vi "save channels to raw bin files.vi"(8 "frame number in":i32, 9 "last frame":bool, 10 "image data in (SGL)":sgl[][](array[numeric]), 11 "image data in (U16)":u16[][](array[numeric])) -> ()   [LabVIEW 2012]
uses:
  Custom Controls/file format type def.ctl
  GFG/GFGpathGet.vi
  GFG/GFG library.lvlib
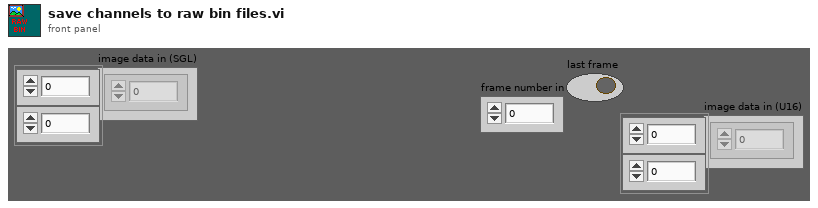
[diagram p1: front panel]
types:
  T1 = enum16{"open", "replace", "create", "open or create", "replace or create", "replace or create with confirmation"}
  T2 = typedef "file format type def.ctl" = enum16{"16bit raw", "32bit raw", "16bit multi-tiff (interleave)", "16bit multi-tiff (separate)", "16bit multi-tiff (stacked)", "32bit multi-tiff (interleave)", "32bit multi-tiff (separate)", "32bit multi-tiff (stacked)", "16bit tiff series (interleave)", "16bit tiff series (separate)", "16bit tiff series (stacked)", "32bit tiff series (interleave)", "32bit tiff series (separate)", "32bit tiff series (stacked)"}
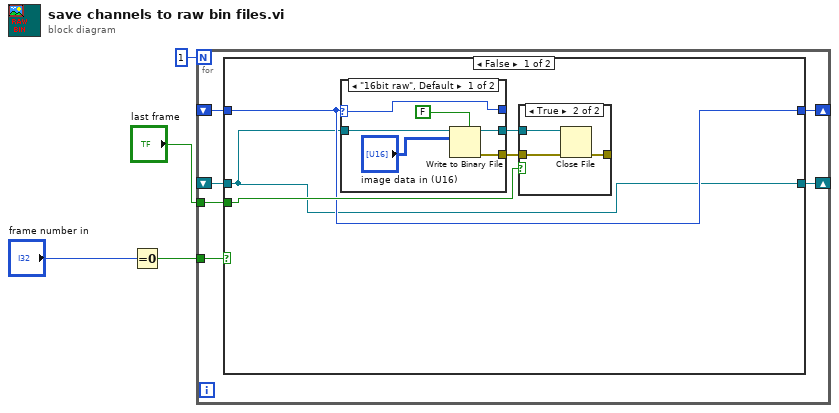
[diagram p0: block diagram]
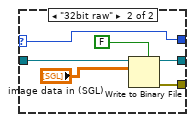
[diagram p3: hidden frame]
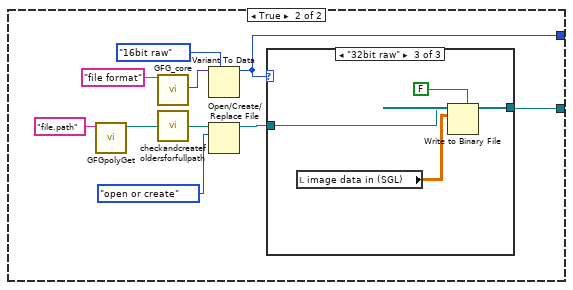
[diagram p4: hidden frame]
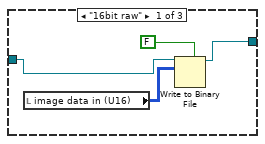
[diagram p5: hidden frame]
diagram:
  n1 = Equal To 0?(x="frame number in") -> (x = 0?=w3:bool)
  n2 = for {
    N: 1 -> [_]
    tunnel: w3 -> [w10]
    shift-right: [w9] -> _
    shift-left: _ -> [w8]
    shift-right: [w7] -> _
    shift-left: _ -> [w6]
    tunnel: "last frame" -> [w5]
    n3 = case shown="False" w10 {
      tunnel: w6 -> [w12 _]
      tunnel: [w11 w32] -> w9
      tunnel: w8 -> [w11 _]
      tunnel: [w12 w38] -> w7
      tunnel: w5 -> [w15 _]
      frame False {
        n4 = case shown="\"16bit raw\", Default" w12 {
          selector: w12 -> [w22 w28]
          tunnel: w11 -> [w24 w30]
          tunnel: [w23 w29] -> w13
          tunnel: [w22 w28] -> _
          tunnel: [w21 w27] -> w14
          frame "16bit raw", Default {
            n5 = Write to Binary File(file (use dialog)=w24, data="image data in (U16)", 5:FALSE ("prepend array or string size? (T)")) -> (refnum out=w21:refnum<file>, error out=w23:errorcluster)  [unwired: 3 in, 1 out]
          }
          frame "32bit raw" {
            n6 = Write to Binary File(file (use dialog)=w30, data="image data in (SGL)", 5:FALSE ("prepend array or string size? (T)")) -> (refnum out=w27:refnum<file>, error out=w29:errorcluster)  [unwired: 3 in, 1 out]
          }
        }
        n7 = case shown="True" w15 {
          tunnel: w14 -> [_ w19]
          tunnel: w13 -> [w16 w18]
          tunnel: [w16 w17] -> _
          frame False {
          }
          frame True {
            n8 = Close File(refnum=w19, error in=w18) -> (error out=w17:errorcluster)  [unwired: 1 out]
          }
        }
      }
      frame True {
        n9 = call-poly "GFGpolyGet.vi"("Variable Name in"="file.path") -> ("Path"=w36:path)  [unwired: 9 in, 1 out]
        n10 = call "GFG_core.vi"("Variable Name in"="file format") -> ("Variant Out"=w40:variant)  [unwired: 12 in, 6 out]
        n11 = call "checkandcreatefoldersforfullpath.vi"("Path IN"=w36) -> ("Path OUT"=w35:path)  [unwired: 4 in]
        n12 = Variant To Data(type=file_format_type_def."16bit raw" ("file format"), Variant=w40) -> (data=w38:T2)  [unwired: 1 in, 1 out]
        n13 = Open/Create/Replace File(file path (use dialog)=w35, operation (0:open)=T1."open or create") -> (refnum out=w33:refnum<file>)  [unwired: 4 in, 2 out]
        n14 = case shown="\"32bit raw\"" w38 {
          tunnel: w33 -> [w44 w46 w49]
          tunnel: [w43 w46 w48] -> w32
          frame "16bit raw" {
            n15 = local read "image data in (U16)"() -> (w42:u16[][])
            n16 = Write to Binary File(file (use dialog)=w44, data=w42, 5:FALSE ("prepend array or string size? (T)")) -> (refnum out=w43:refnum<file>)  [unwired: 3 in, 2 out]
          }
          frame Default {
          }
          frame "32bit raw" {
            n17 = local read "image data in (SGL)"() -> (w47:sgl[][])
            n18 = Write to Binary File(file (use dialog)=w49, data=w47, 5:FALSE ("prepend array or string size? (T)")) -> (refnum out=w48:refnum<file>)  [unwired: 3 in, 2 out]
          }
        }
      }
    }
  }
